vi "Get Record Parameters from Host.vi"(11 "Record Parameters":T3) -> (2 "Acquisition Parameters":T1, 3 "Buffer Parameters":T2)   [LabVIEW 2012]
uses:
  Circular Storage/Buffer Parameters.ctl
  Acquisition Parameters.ctl
  <vilib>/rvi/FXPMathLib/basic elements/FxpDiscreteDelay/XNode/nifxpmath_DiscreteDelay.xnode
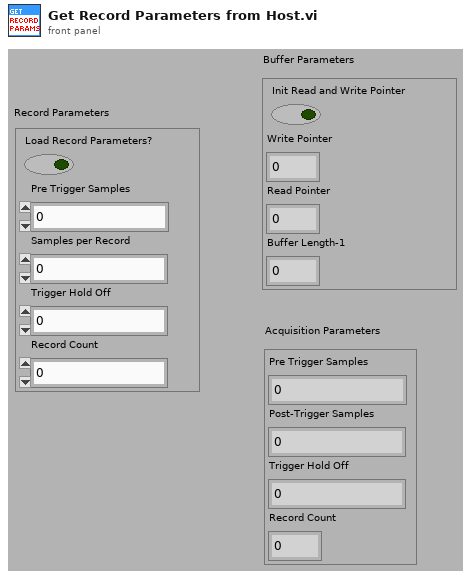
[diagram p1: front panel]
types:
  T1 = typedef "Acquisition Parameters.ctl" = cluster{"Pre Trigger Samples":u16, "Post-Trigger Samples":u16, "Trigger Hold Off":u16, "Record Count":u16}
  T2 = typedef "Buffer Parameters.ctl" = cluster{"Init Read and Write Pointer":bool, "Write Pointer":u16, "Read Pointer":u16, "Buffer Length-1":u16}
  T3 = cluster{"Load Record Parameters?":bool, "Pre Trigger Samples":u16, "Samples per Record":u16, "Trigger Hold Off":u16, "Record Count":u16}
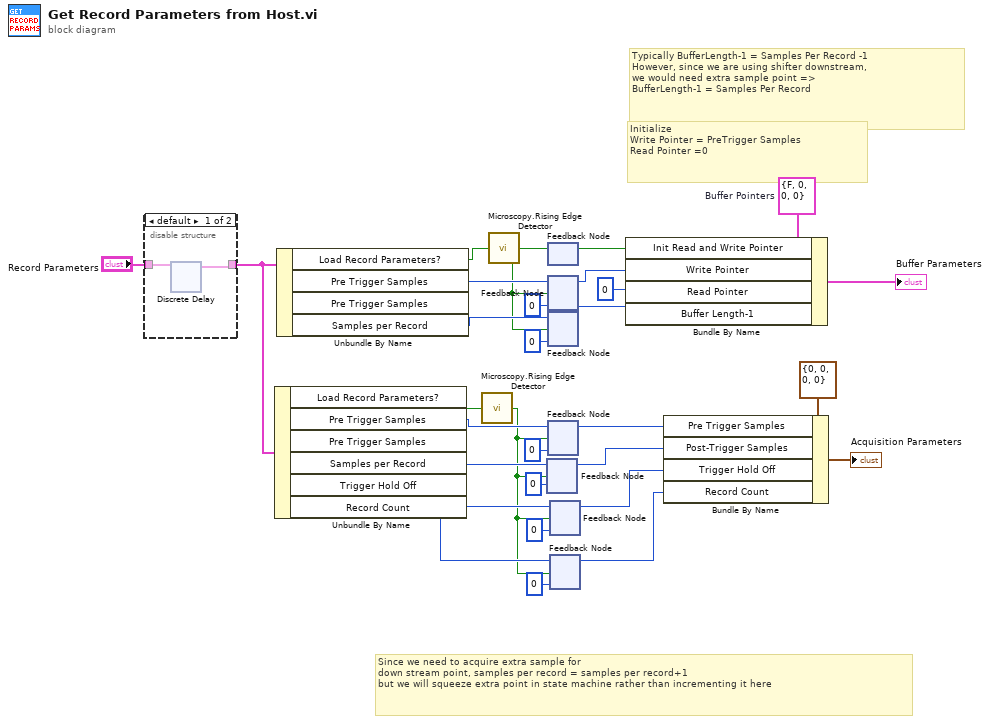
[diagram p0: block diagram]
diagram:
  w30 = T2 {"Init Read and Write Pointer"=FALSE, "Write Pointer"=0, "Read Pointer"=0, "Buffer Length-1"=0}  # Buffer Pointers
  # "Typically BufferLength-1 = Samples Per Record -1\nHowever, since we are using shifter downstream,\nwe would need extra sample point =>\nBufferLength-1 = Samples Per Record"
  # "Since we need to acquire extra sample for \ndown stream point, samples per record = samples per record+1\nbut we will squeeze extra point in state machine rather than incrementing it here"
  # "Initialize \nWrite Pointer = PreTrigger Samples\nRead Pointer =0"
  n1 = disable-structure shown="default" {
    disable-tunnel: "Record Parameters" -> [w32 w33]
    disable-tunnel: [w31 w33] -> w5
    frame condition #0 {
      n2 = xnode "Discrete Delay"("D"=w32) -> ("Q"=w31:T3)
    }
    frame condition #1 (active) {
    }
  }
  n3 = Unbundle By Name(w5) -> ("Load Record Parameters?"=w18:bool, "Pre Trigger Samples"=w17:u16, "Samples per Record"=w16:u16, "Trigger Hold Off"=w7:u16, "Record Count"=w3:u16)  [unwired: 1 out]
  n4 = Unbundle By Name(w5) -> ("Load Record Parameters?"=w27:bool, "Pre Trigger Samples"=w26:u16, "Samples per Record"=w25:u16)  [unwired: 1 out]
  n5 = call "Microscopy.Rising Edge Detector.vi"("signal"=w18) -> ("edge detected"=w2:bool)  [unwired: 14 in]
  n6 = call "Microscopy.Rising Edge Detector.vi"("signal"=w27) -> ("edge detected"=w23:bool)  [unwired: 14 in]
  n7 = feedback #1(u16 0 ("Samples per Record")) -> (w15:u16)
  n8 = feedback-in #1(w16, w2) -> ()
  n9 = feedback-in #2(w23) -> ()
  n10 = feedback #2() -> (w21:bool)  [unwired: 1 in]
  n11 = feedback-in #3(w26, w23) -> ()
  n12 = feedback #3(u16 0 ("Pre Trigger Samples")) -> (w22:u16)
  n13 = feedback #4(u16 0 ("Samples per Record")) -> (w24:u16)
  n14 = feedback-in #4(w25, w23) -> ()
  n15 = feedback #5(u16 0 ("Pre Trigger Samples")) -> (w14:u16)
  n16 = feedback-in #5(w17, w2) -> ()
  n17 = feedback #6(u16 0 ("Samples per Record")) -> (w6:u16)
  n18 = feedback-in #6(w7, w2) -> ()
  n19 = feedback #7(u16 0 ("Samples per Record")) -> (w1:u16)
  n20 = feedback-in #7(w3, w2) -> ()
  n21 = Bundle By Name(cluster=w30, "Init Read and Write Pointer"=w21, "Write Pointer"=w22, "Read Pointer"=u16 0, "Buffer Length-1"=w24) -> (→"Buffer Parameters":T2)
  n22 = Bundle By Name(cluster=T1 {"Pre Trigger Samples"=0, "Post-Trigger Samples"=0, "Trigger Hold Off"=0, "Record Count"=0} ("Acquisition Parameters"), "Pre Trigger Samples"=w14, "Post-Trigger Samples"=w15, "Trigger Hold Off"=w6, "Record Count"=w1) -> (→"Acquisition Parameters":T1)
